vi "Ball Steer.vi"(1 "Reinit?":bool, 2 "Manual Steer":dbl) -> (0 "Steer Amount":dbl)   [LabVIEW 2013]
uses:
  Common Code/Change Detect Boolean.vi
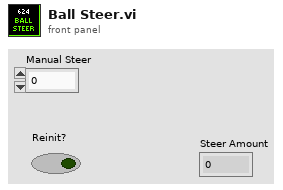
[diagram p1: front panel]
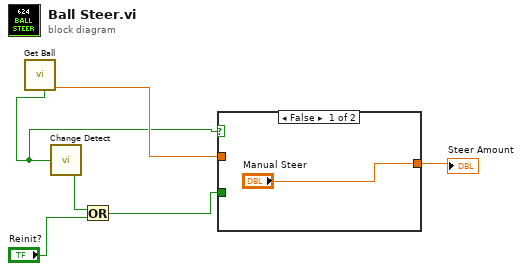
[diagram p0: block diagram]
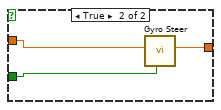
[diagram p2: hidden frame]
diagram:
  n1 = call "Get Ball.vi"() -> ("Field Relative X"=w2:dbl, "Ball Found?"=w1:bool)  [unwired: 8 in, 2 out]
  n2 = call-poly "Change Detect.vi"("In"=w1) -> ("Changed?"=w6:bool)
  n3 = Or(x=w6, y="Reinit?") -> (x .or. y?=w4:bool)
  n4 = case shown="False" w1 {
    tunnel: w4 -> [_ w9]
    tunnel: ["Manual Steer" w10] -> w3
    tunnel: w2 -> [_ w8]
    frame False {
    }
    frame True {
      n5 = call "Gyro Steer.vi"("reinitialize? (F)"=w9, "Target Angle"=w8) -> ("Steering Out"=w10:dbl)  [unwired: 8 in, 1 out]
    }
  }
  "Steer Amount" <- w3
